vi "load_xml.vi"(8 "error in":errorcluster, 10 "child node in":refnum<k20>, 11 "PI_Piezo (in)":refnum<class "PI_Piezo.lvclass">) -> (0 "error out":errorcluster, 2 "child node out":refnum<k20>, 3 "PI_Piezo":refnum<class "PI_Piezo.lvclass">)   [LabVIEW 2013, in "PI_Piezo.lvclass"]
doc: "Loads analog output settings from xml. Expected format:\n\n<Enable>%b</Enable>\n<PhysicalChannel>%s</PhysicalChannel>\n<MinimumValue>%f</MinimumValue>\n<MaximumValue>%f</MaximumValue>\n<SamplesPerSecond>%f</SamplesPerSecond>\n<TotalAOTime units=\"seconds\">%s</TotalAOTime>\n<AnalogOutputEquations>\n%s</AnalogOutputEquations>\n<StartTrigger.WaitForStartTrigger>%b</StartTrigger.WaitForStartTrigger\n<StartTrigger.source>%s</StartTrigger.source>\n<StartTrigger.edge>%s</StartTrigger.edge>\n\nMTL 2012 Dec 31"
uses:
  PI_Piezo.lvclass
  PI_Piezo.lvclass/PI_Piezo.ctl
  piezo_controller.ctl
  piezo_channel.ctl
  Globals.vi
  <vilib>/xml/Close Reference(Node).vi
  <resource>/objmgr/DOMUserDefRef.rc
  <vilib>/xml/NI_XML.lvlib
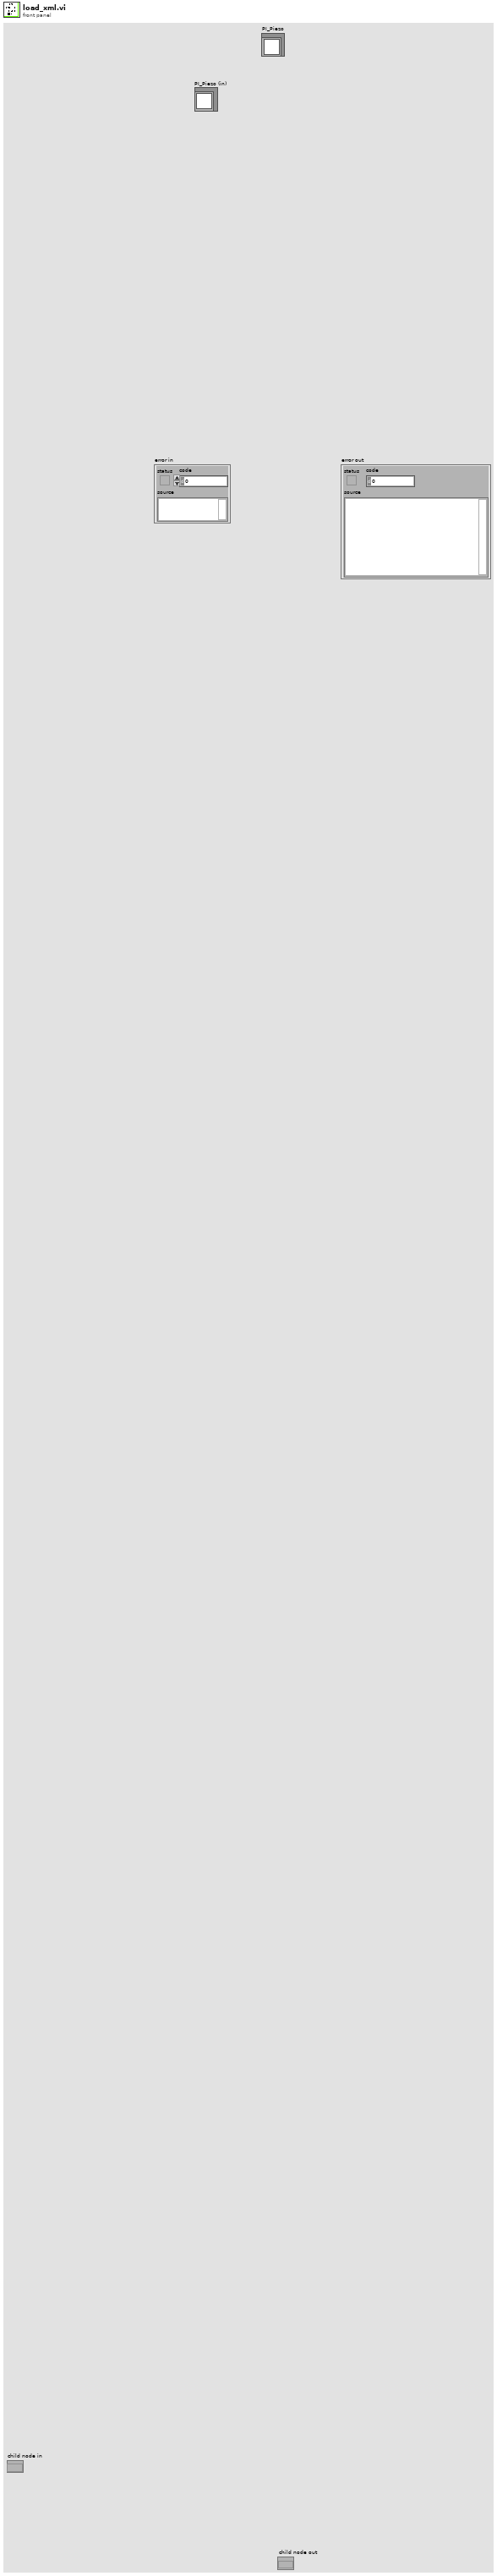
[diagram p1: front panel]
types:
  T1 = typedef "PI_Piezo.lvclass/piezo_channel.ctl" = cluster{"Servo":bool, "Set Position":dbl}
  T2 = typedef "PI_Piezo.lvclass/settings.ctl" = cluster{"Enable":bool, "Array of Piezo Controllers":T3[]}
  T3 = typedef "PI_Piezo.lvclass/piezo_controller.ctl" = cluster{"Enable":bool, "Serial No.":string, "Array of Piezo Channels":T1[]}
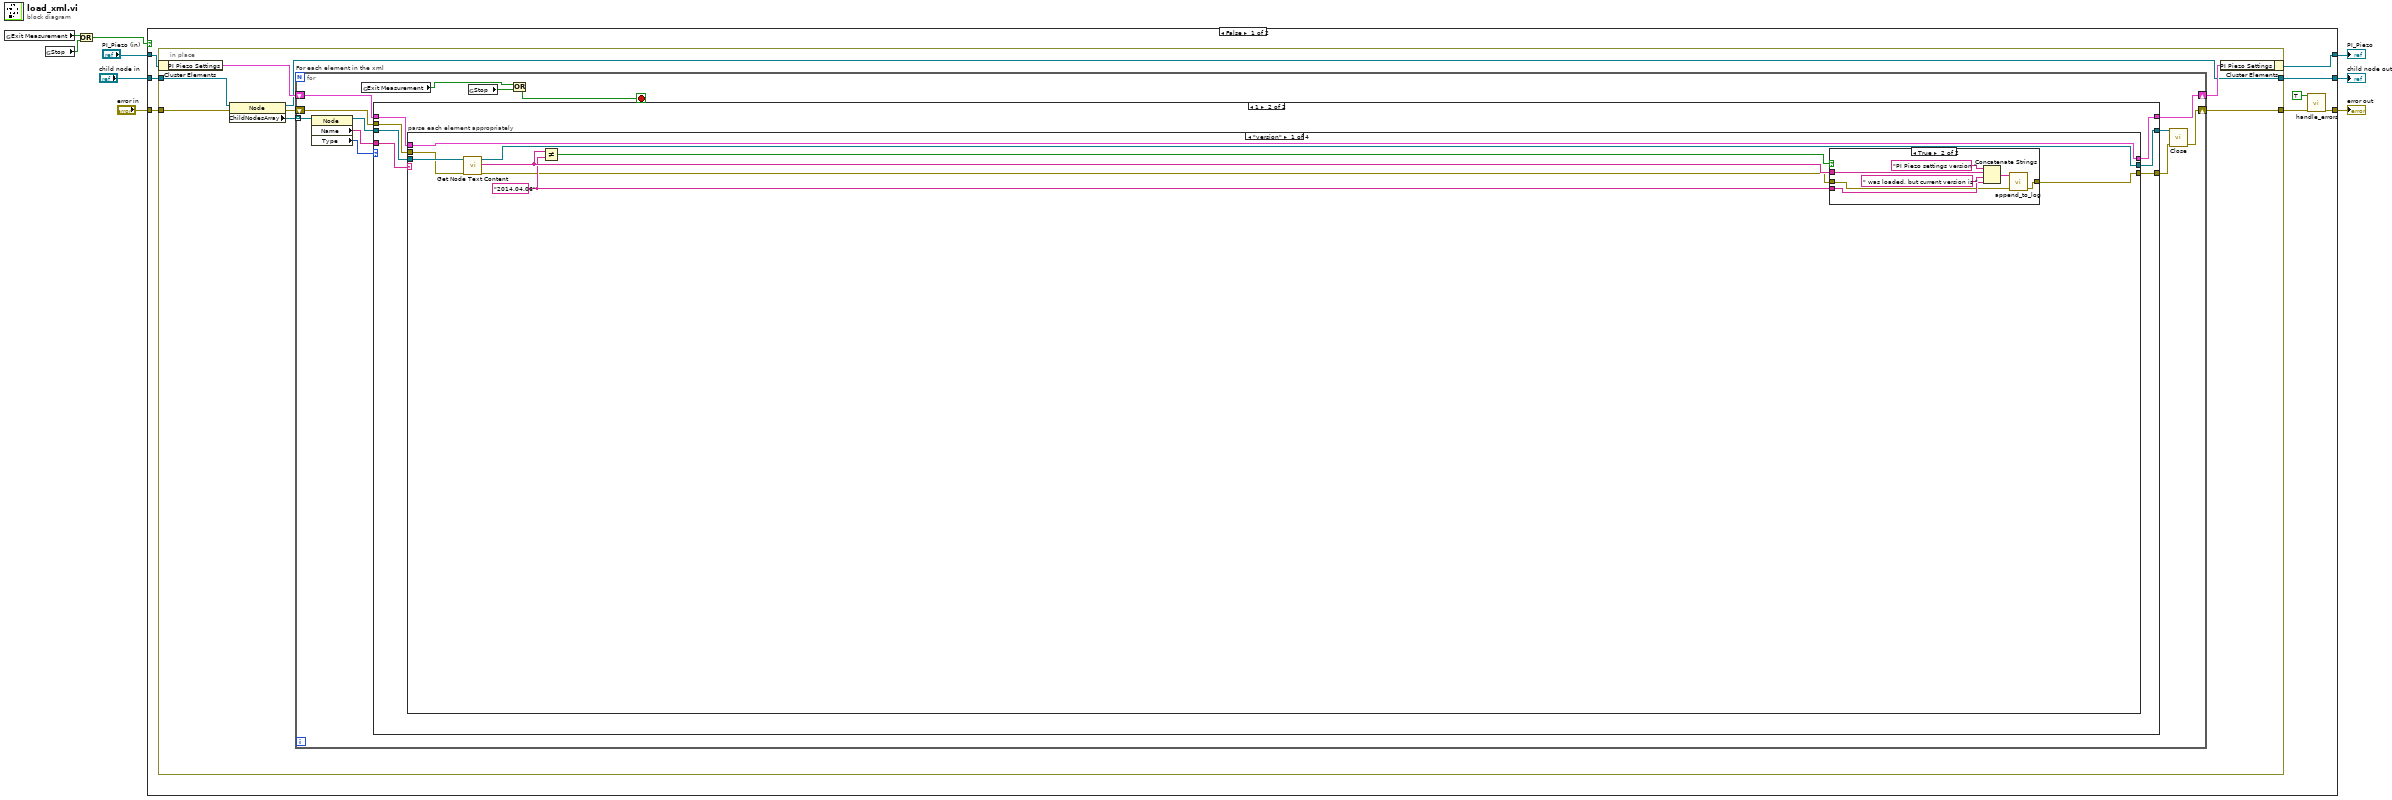
[diagram p0: block diagram]
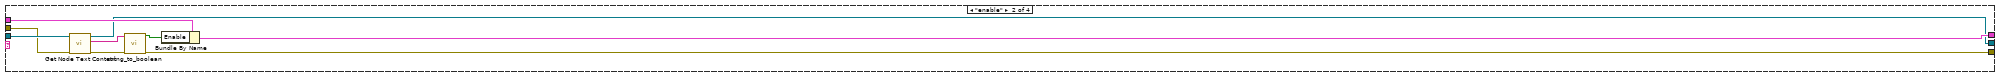
[diagram p4: hidden frame]
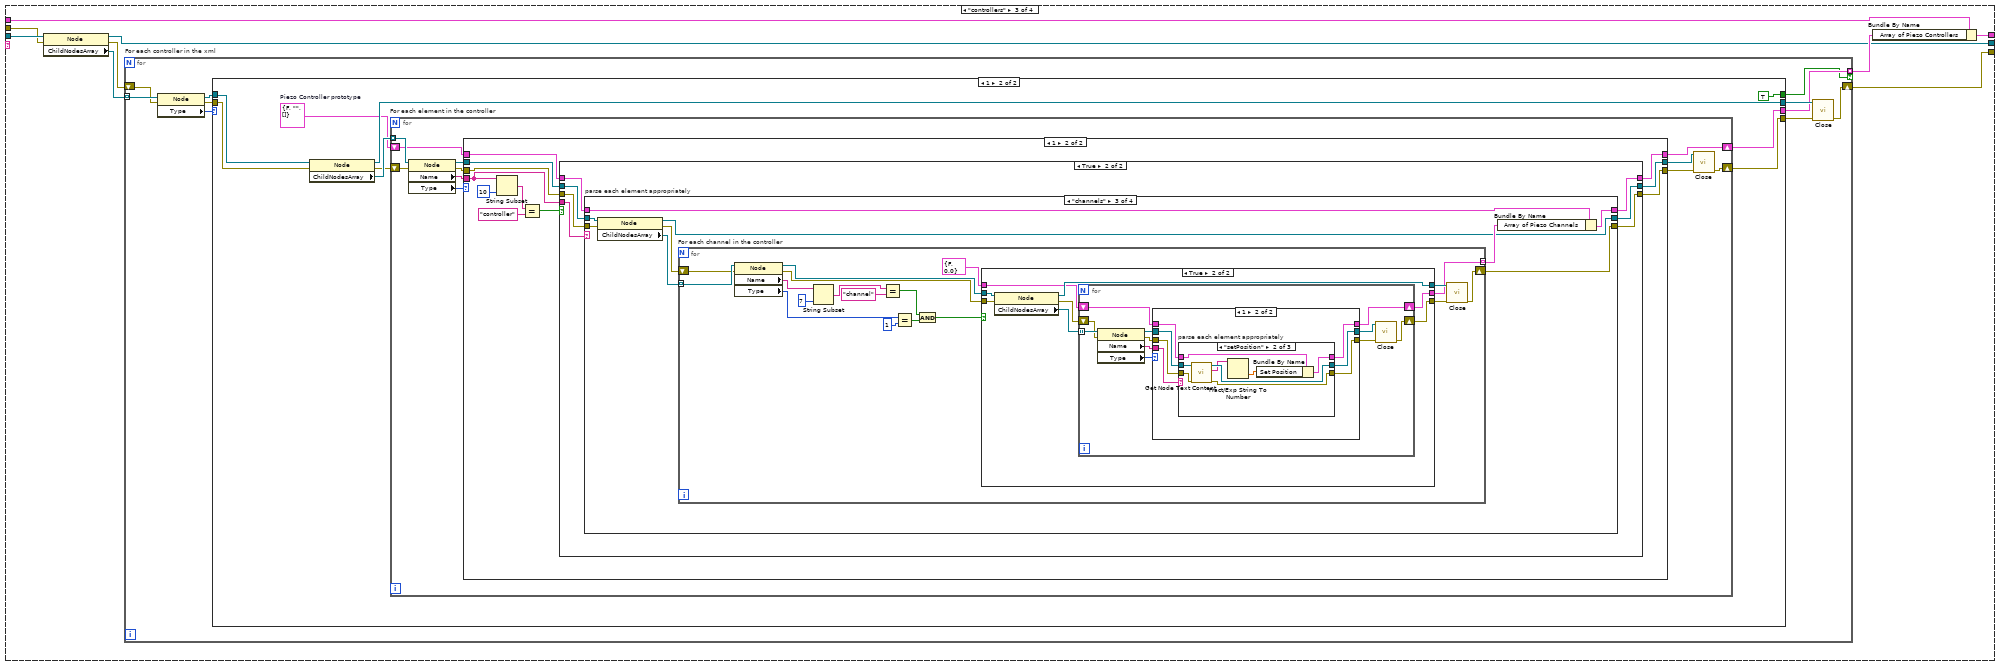
[diagram p5: hidden frame]
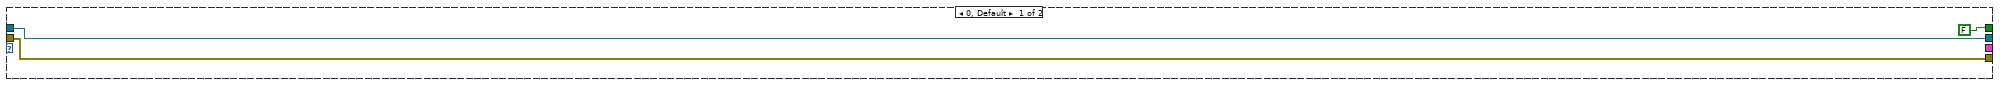
[diagram p6: hidden frame]
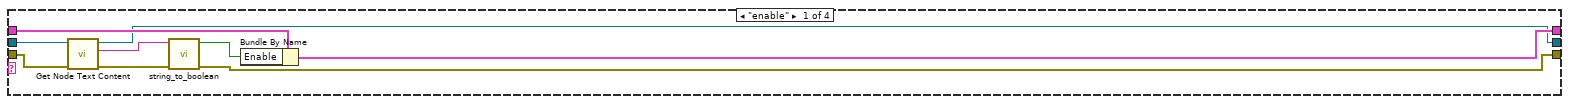
[diagram p9: hidden frame]
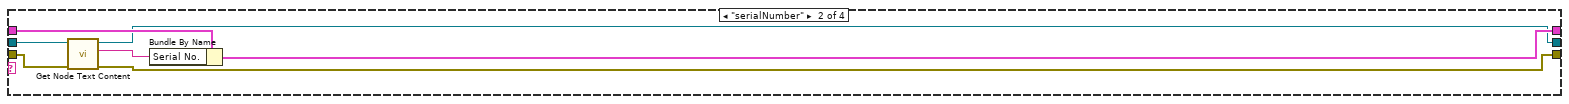
[diagram p10: hidden frame]
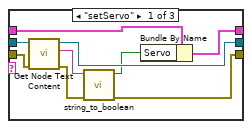
[diagram p13: hidden frame]
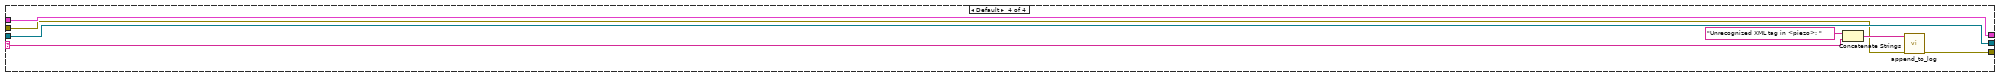
[diagram p16: hidden frame]
diagram:
  n1 = global read "Globals.vi" "Exit Measurement"() -> (w3:bool)
  n2 = global read "Globals.vi" "Stop"() -> (w2:bool)
  n3 = Or(x=w3, y=w2) -> (x .or. y?=w1:bool)
  n4 = case shown="False" w1 {
    tunnel: "PI_Piezo (in)" -> [w17 w246]
    tunnel: [w16 w246] -> w8
    tunnel: [w15 w248] -> w7
    tunnel: "error in" -> [w12 w248]
    tunnel: "child node in" -> [w11 w247]
    tunnel: [w10 w247] -> w4
    frame False {
      n5 = in-place {
        in-place-border: [w21] -> w14
        in-place-border: w12 -> [w20]
        in-place-border: w11 -> [w18]
        in-place-border: [w19] -> w10
        n6 = in-place-cluster #1(w17) -> ("PI Piezo Settings"=w23:T2)
        n7 = property class="Node"(reference=w18, error in=w20) -> (reference out=w19:refnum<k20>, error out=w24:errorcluster, "ChildNodesArray"=w25:refnum<k20>[])
        n8 = for "For each element in the xml" {
          tunnel: w25 -> [w38] mode=indexing
          shift-right: [w32] -> w21
          shift-left: w24 -> [w35]
          shift-right: [w30] -> w22
          shift-left: w23 -> [w31]
          stop <- w26 stop-if-true
          n9 = property class="Node"(reference=w38) -> (reference out=w37:refnum<k20>, "Name"=w36:string, "Type"=w29:i32)  [unwired: 1 in, 1 out]
          n10 = global read "Globals.vi" "Exit Measurement"() -> (w28:bool)
          n11 = case shown="1" w29 {
            tunnel: w37 -> [w41 w48]
            tunnel: w36 -> [_ w47]
            tunnel: w35 -> [w40 w46]
            tunnel: [w41 w45] -> w34
            tunnel: [w40 w44] -> w33
            tunnel: w31 -> [w39 w43]
            tunnel: [w39 w42] -> w30
            frame Default {
            }
            frame 1 {
              n12 = case "parse each element appropriately" shown="\"version\"" w47 {
                selector: w47 -> [_ _ _ w239]
                tunnel: [w50 w68 w75 w245] -> w45
                tunnel: w48 -> [w53 w74 w79 w245]
                tunnel: w46 -> [w52 w73 w77 w241]
                tunnel: [w51 w67 w83 w240] -> w44
                tunnel: w43 -> [w49 w70 w81 w244]
                tunnel: [w49 w69 w82 w244] -> w42
                frame "version" {
                  w55 = "2014.04.06" ("y")
                  n13 = call <vilib>:"Get Node Text Content.vi"("error in (no error)"=w52, "node in"=w53) -> ("error out"=w54:errorcluster, "node text"=w56:string, "node out"=w50:refnum<k20>)  [unwired: 7 in]
                  n14 = Not Equal?(x=w56, y=w55) -> (x != y?=w57:bool)
                  n15 = case shown="True" w57 {
                    tunnel: w56 -> [_ w64]
                    tunnel: w55 -> [_ w62]
                    tunnel: w54 -> [w58 w60]
                    tunnel: [w58 w59] -> w51
                    frame False {
                    }
                    frame True {
                      n16 = Concatenate Strings("PI Piezo settings version " ("string"), w64, " was loaded, but current version is " ("string"), w62) -> (w61:string)
                      n17 = call "append_to_log.vi"("error in"=w60, "string"=w61) -> ("error out"=w59:errorcluster)  [unwired: 9 in]
                    }
                  }
                }
                frame "enable" {
                  n18 = call <vilib>:"Get Node Text Content.vi"("error in (no error)"=w73, "node in"=w74) -> ("error out"=w71:errorcluster, "node text"=w72:string, "node out"=w68:refnum<k20>)  [unwired: 7 in]
                  n19 = call "string_to_boolean.vi"("error in"=w71, "string"=w72) -> ("error out"=w67:errorcluster, "boolean"=w66:bool)  [unwired: 8 in]
                  n20 = Bundle By Name(cluster=w70, "Enable"=w66) -> (w69:T2)
                }
                frame "controllers" {
                  n21 = property class="Node"(reference=w79, error in=w77) -> (reference out=w75:refnum<k20>, error out=w76:errorcluster, "ChildNodesArray"=w78:refnum<k20>[])
                  n22 = for "For each controller in the xml" {
                    tunnel: w78 -> [w88] mode=indexing
                    shift-right: [w91] -> w83
                    shift-left: w76 -> [w85]
                    tunnel: [w90] -> w80 mode=indexing if=w89
                    n23 = property class="Node"(reference=w88, error in=w85) -> (reference out=w87:refnum<k20>, error out=w84:errorcluster, "Type"=w86:i32)
                    n24 = case shown="1" w86 {
                      tunnel: w87 -> [w96 w105]
                      tunnel: w84 -> [w94 w104]
                      tunnel: [w96 w101] -> w93
                      tunnel: [w94 w100] -> w92
                      tunnel: [_ w99] -> w90
                      tunnel: [FALSE TRUE] -> w89
                      frame 0, Default {
                      }
                      frame 1 {
                        w98 = T3 {"Enable"=FALSE, "Serial No."="", "Array of Piezo Channels"=[]}  # Piezo Controller prototype
                        n25 = property class="Node"(reference=w105, error in=w104) -> (reference out=w101:refnum<k20>, error out=w102:errorcluster, "ChildNodesArray"=w103:refnum<k20>[])
                        n26 = for "For each element in the controller" {
                          shift-right: [w109] -> w100
                          shift-left: w102 -> [w113]
                          tunnel: w103 -> [w116] mode=indexing
                          shift-right: [w107] -> w99
                          shift-left: w98 -> [w108]
                          n27 = property class="Node"(reference=w116, error in=w113) -> (reference out=w111:refnum<k20>, error out=w114:errorcluster, "Name"=w115:string, "Type"=w106:i32)
                          n28 = case shown="1" w106 {
                            tunnel: w115 -> [_ w125]
                            tunnel: w114 -> [w118 w130]
                            tunnel: [w119 w120] -> w112
                            tunnel: w111 -> [w119 w129]
                            tunnel: [w118 w128] -> w110
                            tunnel: w108 -> [w117 w127]
                            tunnel: [w117 w126] -> w107
                            frame Default {
                            }
                            frame 1 {
                              n29 = String Subset(string=w125, length (rest)=10 ("length (rest)")) -> (substring=w123:string)  [unwired: 1 in]
                              n30 = Equal?(x=w123, y="controller") -> (x = y?=w121:bool)
                              n31 = case shown="True" w121 {
                                tunnel: w125 -> [_ w140]
                                tunnel: w130 -> [w132 w139]
                                tunnel: w129 -> [w133 w137]
                                tunnel: [w132 w136] -> w128
                                tunnel: w127 -> [w131 w135]
                                tunnel: [w131 w134] -> w126
                                tunnel: [w133 w138] -> w120
                                frame False {
                                }
                                frame True {
                                n32 = case "parse each element appropriately" shown="\"channels\"" w140 {
                                tunnel: w139 -> [w148 w155 w159 w238]
                                tunnel: [w141 w150 w165 w238] -> w136
                                tunnel: [w145 w151 w157 w237] -> w138
                                tunnel: w137 -> [w149 w156 w161 w237]
                                tunnel: w135 -> [w147 w154 w163 w236]
                                tunnel: [w146 w153 w164 w236] -> w134
                                frame "enable" {
                                n33 = call <vilib>:"Get Node Text Content.vi"("error in (no error)"=w148, "node in"=w149) -> ("error out"=w142:errorcluster, "node text"=w144:string, "node out"=w145:refnum<k20>)  [unwired: 7 in]
                                n34 = call "string_to_boolean.vi"("error in"=w142, "string"=w144) -> ("error out"=w141:errorcluster, "boolean"=w143:bool)  [unwired: 8 in]
                                n35 = Bundle By Name(cluster=w147, "Enable"=w143) -> (w146:T3)
                                }
                                frame "serialNumber" {
                                n36 = call <vilib>:"Get Node Text Content.vi"("error in (no error)"=w155, "node in"=w156) -> ("error out"=w150:errorcluster, "node text"=w152:string, "node out"=w151:refnum<k20>)  [unwired: 7 in]
                                n37 = Bundle By Name(cluster=w154, "Serial No."=w152) -> (w153:T3)
                                }
                                frame "channels" {
                                n38 = property class="Node"(reference=w161, error in=w159) -> (reference out=w157:refnum<k20>, error out=w158:errorcluster, "ChildNodesArray"=w160:refnum<k20>[])
                                n39 = for "For each channel in the controller" {
                                shift-right: [w183] -> w165
                                shift-left: w158 -> [w178]
                                tunnel: w160 -> [w179] mode=indexing
                                tunnel: [w181] -> w162 mode=indexing
                                n40 = property class="Node"(reference=w179, error in=w178) -> (reference out=w177:refnum<k20>, error out=w167:errorcluster, "Name"=w176:string, "Type"=w170:i32)
                                n41 = String Subset(string=w176, length (rest)=7 ("length (rest)")) -> (substring=w174:string)  [unwired: 1 in]
                                n42 = Equal?(x=w174, y="channel" ("XPath expression")) -> (x = y?=w171:bool)
                                n43 = Equal?(x=w170, y=1) -> (x = y?=w168:bool)
                                n44 = And(x=w171, y=w168) -> (x .and. y?=w172:bool)
                                n45 = case shown="True" w172 {
                                tunnel: w177 -> [w185 w194]
                                tunnel: w167 -> [w186 w193]
                                tunnel: [w185 w192] -> w182
                                tunnel: [w184 w189] -> w181
                                tunnel: [w186 w188] -> w180
                                tunnel: T1 {"Servo"=FALSE, "Set Position"=0.0} ("Piezo Channel") -> [w184 w187]
                                frame False {
                                }
                                frame True {
                                n46 = property class="Node"(reference=w194, error in=w193) -> (reference out=w192:refnum<k20>, error out=w190:errorcluster, "ChildNodesArray"=w191:refnum<k20>[])
                                n47 = for {
                                tunnel: w191 -> [w205] mode=indexing
                                shift-right: [w199] -> w188
                                shift-left: w190 -> [w203]
                                shift-right: [w196] -> w189
                                shift-left: w187 -> [w197]
                                n48 = property class="Node"(reference=w205, error in=w203) -> (reference out=w201:refnum<k20>, error out=w202:errorcluster, "Name"=w204:string, "Type"=w195:i32)
                                n49 = case shown="1" w195 {
                                tunnel: w204 -> [_ w215]
                                tunnel: w202 -> [w207 w214]
                                tunnel: w201 -> [w208 w213]
                                tunnel: [w208 w212] -> w200
                                tunnel: [w207 w211] -> w198
                                tunnel: w197 -> [w206 w210]
                                tunnel: [w206 w209] -> w196
                                frame Default {
                                }
                                frame 1 {
                                n50 = case "parse each element appropriately" shown="\"setPosition\"" w215 {
                                tunnel: [w219 w232 w235] -> w211
                                tunnel: [w224 w231 w233] -> w212
                                tunnel: [w223 w230 w234] -> w209
                                tunnel: w214 -> [w222 w228 w235]
                                tunnel: w213 -> [w221 w229 w233]
                                tunnel: w210 -> [w218 w227 w234]
                                frame "setServo" {
                                n51 = call <vilib>:"Get Node Text Content.vi"("error in (no error)"=w222, "node in"=w221) -> ("error out"=w220:errorcluster, "node text"=w216:string, "node out"=w224:refnum<k20>)  [unwired: 7 in]
                                n52 = call "string_to_boolean.vi"("error in"=w220, "string"=w216) -> ("error out"=w219:errorcluster, "boolean"=w217:bool)  [unwired: 8 in]
                                n53 = Bundle By Name(cluster=w218, "Servo"=w217) -> (w223:T1)
                                }
                                frame "setPosition" {
                                n54 = call <vilib>:"Get Node Text Content.vi"("error in (no error)"=w228, "node in"=w229) -> ("error out"=w232:errorcluster, "node text"=w226:string, "node out"=w231:refnum<k20>)  [unwired: 7 in]
                                n55 = Fract/Exp String To Number(string=w226) -> (number=w225:dbl)  [unwired: 3 in, 1 out]
                                n56 = Bundle By Name(cluster=w227, "Set Position"=w225) -> (w230:T1)
                                }
                                frame Default {
                                }
                                }
                                }
                                }
                                n57 = call-poly <vilib>:"Close.vi"("error in (no error)"=w198, "node"=w200) -> ("error out"=w199:errorcluster)  [unwired: 7 in]
                                }
                                }
                                }
                                n58 = call-poly <vilib>:"Close.vi"("error in (no error)"=w180, "node"=w182) -> ("error out"=w183:errorcluster)  [unwired: 7 in]
                                }
                                n59 = Bundle By Name(cluster=w163, "Array of Piezo Channels"=w162) -> (w164:T3)
                                }
                                frame "None", Default {
                                }
                                }
                                }
                              }
                            }
                          }
                          n60 = call-poly <vilib>:"Close.vi"("error in (no error)"=w110, "node"=w112) -> ("error out"=w109:errorcluster)  [unwired: 7 in]
                        }
                      }
                    }
                    n61 = call-poly <vilib>:"Close.vi"("error in (no error)"=w92, "node"=w93) -> ("error out"=w91:errorcluster)  [unwired: 7 in]
                  }
                  n62 = Bundle By Name(cluster=w81, "Array of Piezo Controllers"=w80) -> (w82:T2)
                }
                frame Default {
                  n63 = Concatenate Strings("Unrecognized XML tag in <piezo>: " ("string"), w239) -> (w242:string)
                  n64 = call "append_to_log.vi"("error in"=w241, "string"=w242) -> ("error out"=w240:errorcluster)  [unwired: 9 in]
                }
              }
            }
          }
          n65 = global read "Globals.vi" "Stop"() -> (w27:bool)
          n66 = Or(x=w28, y=w27) -> (x .or. y?=w26:bool)
          n67 = call-poly <vilib>:"Close.vi"("error in (no error)"=w33, "node"=w34) -> ("error out"=w32:errorcluster)  [unwired: 7 in]
        }
        n68 = in-place-cluster #1("PI Piezo Settings"=w22) -> (w16:refnum<class "PI_Piezo.lvclass">)
      }
      n69 = call "handle_errors.vi"("Exit Operation"=TRUE ("Exit Measurement"), "error in (no error)"=w14) -> ("error out"=w15:errorcluster)  [unwired: 13 in]
    }
    frame True {
    }
  }
  "PI_Piezo" <- w8
  "error out" <- w7
  "child node out" <- w4
